vi "SVPO TDMS Write SGL Waveform (1 Ch).vi"(0 "tdms file":refnum<k34>, 1 "write channel properties? (T)":bool=TRUE, 5 "group name in":string="Waveform", 7 "channel name in":string="Channel0", 9 "scaled signal [EU]":waveform(sgl)) -> (4 "tdms file out":refnum<k34>, 6 "group name out":string, 8 "channel name out":string)   [LabVIEW 2017]
doc: "Writes single-precision waveform or scaled array data to the specified .tdms file in a format specific to the polymorphic instance. Use this VI on embedded targets that have limited computational resources. Wire data to the <B>scaled signal [EU]</B> input to determine the polymorphic instance to use or manually select the instance."
uses:
  <vilib>/addons/_NISVFA/_Shared subVIs/Controls/LV Datatypes.ctl
  <vilib>/addons/_NISVFA/_Shared subVIs/Controls/NI Function Type.ctl
  <vilib>/addons/_NISVFA/_Shared subVIs/Controls/NI Function SubType.ctl
  <vilib>/addons/_NISVFA/_Shared subVIs/Controls/svc_X-Axis Units.ctl
  <vilib>/addons/_NISVFA/_Shared subVIs/Controls/svc_Unit Info.ctl
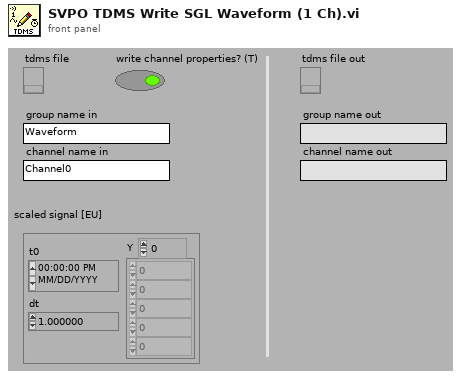
[diagram p1: front panel]
types:
  T1 = typedef "svc_Unit Info.ctl" = cluster{"X-axis label":string, "X-unit string":string, "Y-axis label":string, "Y-unit string":string}
  T2 = typedef "NI Function Type.ctl" = u16
  T3 = typedef "NI Function SubType.ctl" = u16
  T4 = typedef "svc_X-Axis Units.ctl" = u16
  T5 = cluster{"function type":T2, "function subtype":T3, "X-dimension":T4}
  T6 = typedef "LV Datatypes.ctl" = i32
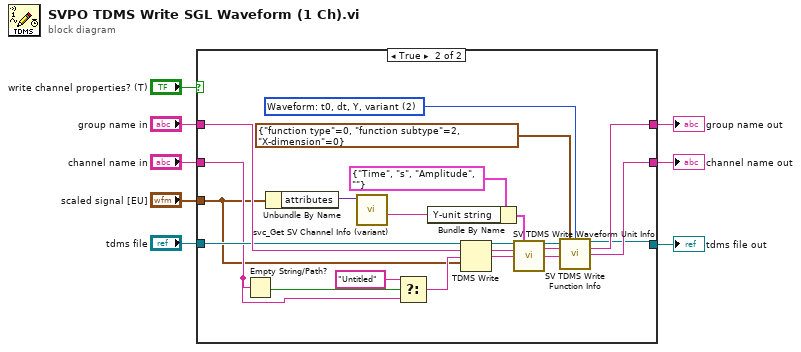
[diagram p0: block diagram]
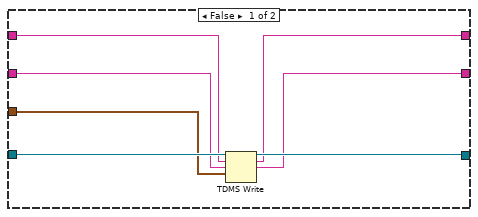
[diagram p2: hidden frame]
diagram:
  n1 = case shown="True" "write channel properties? (T)" {
    tunnel: [w14 w19] -> w8
    tunnel: "channel name in" -> [w10 w31]
    tunnel: "group name in" -> [w11 w37]
    tunnel: "tdms file" -> [w15 w36]
    tunnel: "scaled signal [EU]" -> [w9 w27]
    tunnel: [w13 w20] -> w1
    tunnel: [w12 w21] -> w3
    frame False {
      n2 = TDMS Write(0:w15, 5:w11, 7:w10, 9:w9) -> (4:w14:refnum<k34>, 6:w13:string, 8:w12:string)  [unwired: 2 in, 1 out]
    }
    frame True {
      w26 = T6 2 items=["String"=-2, "Boolean"=-1, "Scalar: y"=0, "Array: Y"=1, "Waveform: t0, dt, Y, variant"=2, "Cluster: x0, dx, Y"=3, "Cluster: X, Y"=4, "Waterfall"=5, "Colormap"=6] ("LabVIEW datatype")
      n3 = Empty String/Path?(string/path=w31) -> (empty?=w32:bool)
      n4 = Unbundle By Name(w27) -> ("attributes"=w28:variant)
      n5 = call <vilib>:"svc_Get SV Channel Info (variant).vi"("attributes"=w28) -> ("unit label"=w16:string)  [unwired: 5 in, 5 out]
      n6 = Select(t="Untitled", s=w32, f=w31) -> (s? t:f=w30:string)
      n7 = Bundle By Name(cluster=T1 {"X-axis label"="Time", "X-unit string"="s", "Y-axis label"="Amplitude", "Y-unit string"=""} ("unit info"), "Y-unit string"=w16) -> (w17:T1)
      n8 = TDMS Write(0:w36, 5:w37, 7:w30, 9:w27) -> (4:w35:refnum<k34>, 6:w34:string, 8:w33:string)  [unwired: 2 in, 1 out]
      n9 = call <vilib>:"SV TDMS Write Waveform Unit Info.vi"("tdms file"=w35, "unit info"=w17, "group name"=w34, "channel name"=w33) -> ("tdms file out"=w24:refnum<k34>, "group name out"=w23:string, "channel name out"=w22:string)  [unwired: 8 in, 1 out]
      n10 = call <vilib>:"SV TDMS Write Function Info.vi"("tdms file in"=w24, "function info"=T5 {"function type"=0, "function subtype"=2, "X-dimension"=0}, "LabVIEW datatype"=w26, "group name"=w23, "channel name"=w22) -> ("tdms file out"=w19:refnum<k34>, "group name out"=w20:string, "channel name out"=w21:string)  [unwired: 7 in, 1 out]
    }
  }
  "tdms file out" <- w8
  "channel name out" <- w3
  "group name out" <- w1
